vi "PQcmdStatus.vi"(8 "error in (no error)":errorcluster, 10 "res":u32) -> (0 "error out":errorcluster, 2 "PQcmdStatus":string)   [LabVIEW 2019, in "libpqlv.lvlib"]
uses:
  libpqlv.lvlib
  libpq.dll
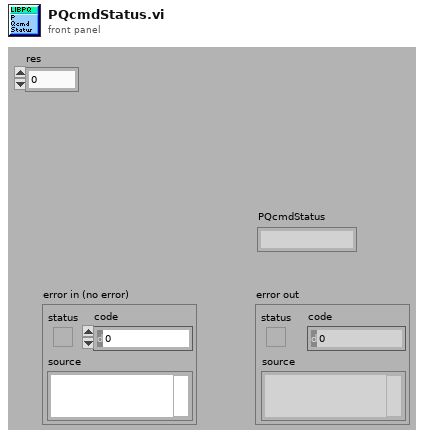
[diagram p1: front panel]
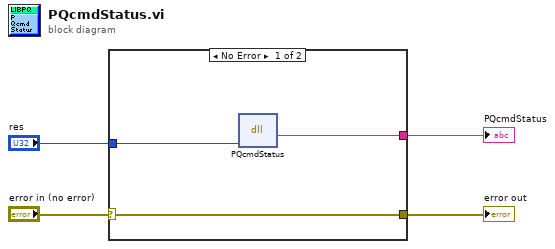
[diagram p0: block diagram]
diagram:
  n1 = case shown="No Error" "error in (no error)" {
    selector: "error in (no error)" -> [w7 w8]
    tunnel: [w7 w8] -> w3
    tunnel: [w6 _] -> w2
    tunnel: "res" -> [w5 _]
    frame No Error {
      n2 = dll-call lib="libpq.*" fn="PQcmdStatus"("res"=w5) -> ("PQcmdStatus"=w6:string)  [unwired: 4 in, 2 out]
    }
    frame Error {
    }
  }
  "PQcmdStatus" <- w2
  "error out" <- w3
